vi "P9P14_Splitt_Cluster.vi"(0 "P9/P14-Magnet-Cluster":T3 {"Magnet Status" items=["MagnetUnknown"=0, "StablePersistent"=1, "WarmingSwitch"=2, "CoolingSwitch"=3, "StableDriven"=4, "Iterating"=5, "Charging"=6, "Discharging"=7, "CurrentError"=8, "MagnetFailure"=15]; "Approach" items=["Linear", "NoOvershoot", "Oscillate"]}) -> (1 "P9/P14-Magnet Status":T2 {"Magnet Status" items=["MagnetUnknown"=0, "StablePersistent"=1, "WarmingSwitch"=2, "CoolingSwitch"=3, "StableDriven"=4, "Iterating"=5, "Charging"=6, "Discharging"=7, "CurrentError"=8, "MagnetFailure"=15]}, 3 "P9/P14-Magnet-Control":T1 {"Approach" items=["Linear", "NoOvershoot", "Oscillate"]})   [LabVIEW 2019]
uses:
  PPMS/P9_P14_Magnet-cluster.ctl
  PPMS/P9P14_Magnet_Status.ctl
  PPMS/P9P14_Magnet_Control.ctl
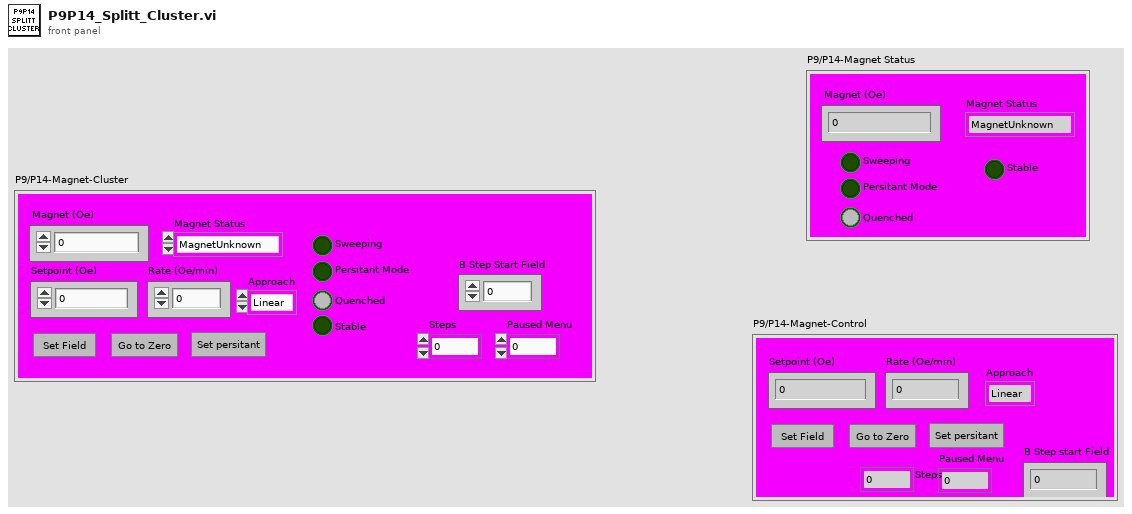
[diagram p1: front panel]
types:
  T1 = typedef "P9P14_Magnet_Control.ctl" = cluster{"Setpoint (Oe)":dbl, "Rate (Oe/min)":dbl, "Set Field":bool, "Go to zero":bool, "Set Persitant/non-pers":bool, "Approach":i32, "Steps":dbl, "Paused Menu":dbl, "B Step start Field":dbl}
  T2 = typedef "P9P14_Magnet_Status.ctl" = cluster{"Magnet (Oe)":dbl, "Magnet Status":i32, "Sweeping":bool, "Quenched":bool, "Persitant Mode ":bool, "Stable":bool}
  T3 = typedef "P9_P14_Magnet-cluster.ctl" = cluster{"Magnet (Oe)":dbl, "Setpoint (Oe)":dbl, "Rate (Oe/min)":dbl, "Set Field":bool, "Go to zero":bool, "Set Persitant/non-pers":bool, "Approach":i32, "Magnet Status":i32, "Sweeping":bool, "Quenched":bool, "Persitant Mode ":bool, "Stable":bool, "Steps":dbl, "Paused Menu":dbl, "B Step Start Field":dbl}
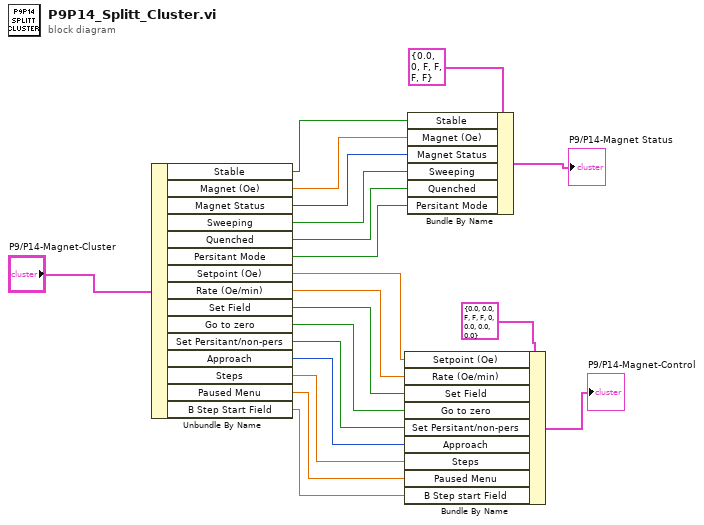
[diagram p0: block diagram]
diagram:
  n1 = Unbundle By Name("P9/P14-Magnet-Cluster") -> ("Stable"=w1:bool, "Magnet (Oe)"=w15:dbl, "Magnet Status"=w14:i32, "Sweeping"=w13:bool, "Quenched"=w12:bool, "Persitant Mode"=w11:bool, "Setpoint (Oe)"=w10:dbl, "Rate (Oe/min)"=w9:dbl, "Set Field"=w8:bool, "Go to zero"=w7:bool, "Set Persitant/non-pers"=w6:bool, "Approach"=w5:i32, "Steps"=w4:dbl, "Paused Menu"=w3:dbl, "B Step Start Field"=w2:dbl)
  n2 = Bundle By Name(cluster=T1 {"Setpoint (Oe)"=0.0, "Rate (Oe/min)"=0.0, "Set Field"=FALSE, "Go to zero"=FALSE, "Set Persitant/non-pers"=FALSE, "Approach"=0, "Steps"=0.0, "Paused Menu"=0.0, "B Step start Field"=0.0} ("P9/P14-Magnet-Control"), "Setpoint (Oe)"=w10, "Rate (Oe/min)"=w9, "Set Field"=w8, "Go to zero"=w7, "Set Persitant/non-pers"=w6, "Approach"=w5, "Steps"=w4, "Paused Menu"=w3, "B Step start Field"=w2) -> (→"P9/P14-Magnet-Control":T1)
  n3 = Bundle By Name(cluster=T2 {"Magnet (Oe)"=0.0, "Magnet Status"=0, "Sweeping"=FALSE, "Quenched"=FALSE, "Persitant Mode "=FALSE, "Stable"=FALSE} ("P9/P14-Magnet Status"), "Stable"=w1, "Magnet (Oe)"=w15, "Magnet Status"=w14, "Sweeping"=w13, "Quenched"=w12, "Persitant Mode"=w11) -> (→"P9/P14-Magnet Status":T2)
